vi "read_params.vi"(8 "error in (no error)":errorcluster, 11 "Perceptron in":refnum<class "Perceptron.lvclass">) -> (0 "error out":errorcluster, 2 "params":T1={"penalty"="l2", "alpha"=0.001, "l1_ratio"=0.15, "fit_intercept"=TRUE, "max_iter"=1000.0, "tol"=0.001, "shuffle"=TRUE, "verbose"=0.0, "n_jobs"=1.0, "random_state"=0.0, "early_stopping"=FALSE, "validation_fraction"=0.1, "n_iter_no_change"=5.0, "class_weight"={"class_weight_type"="None", "class_weight_dict"="{0:1.2,1:0.8,2:1.0}"}, "warm_start"=FALSE}, 3 "Perceptron out":refnum<class "Perceptron.lvclass">)   [LabVIEW 2020, in "Perceptron.lvclass"]
uses:
  Perceptron.lvclass
  Controls/perceptron_params.ctl
  Perceptron.lvclass/Perceptron.ctl
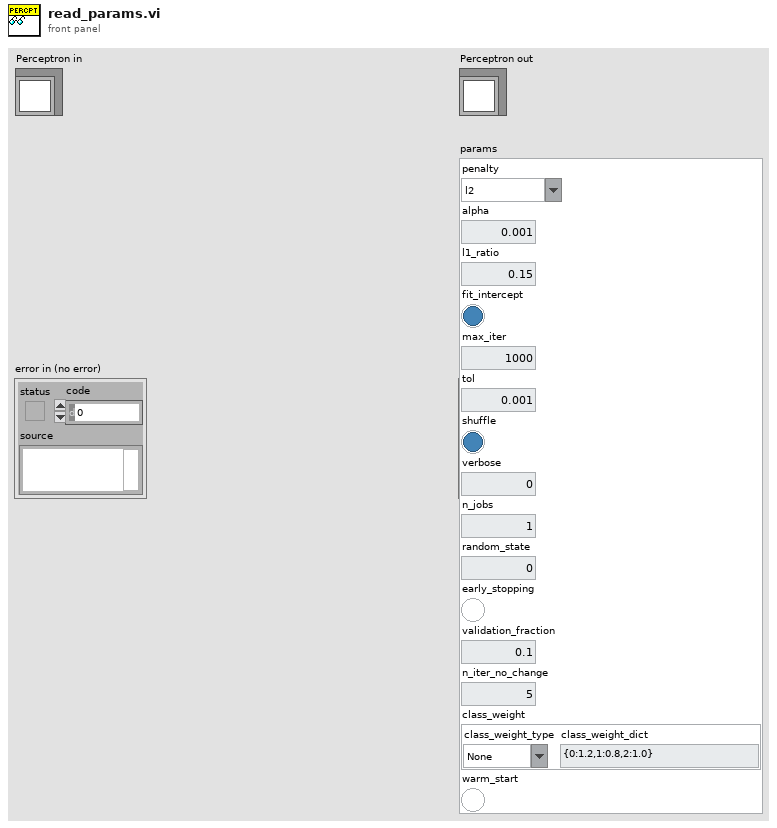
[diagram p1: front panel]
types:
  T1 = typedef "perceptron_params.ctl" = cluster{"penalty":string, "alpha":dbl, "l1_ratio":dbl, "fit_intercept":bool, "max_iter":dbl, "tol":dbl, "shuffle":bool, "verbose":dbl, "n_jobs":dbl, "random_state":dbl, "early_stopping":bool, "validation_fraction":dbl, "n_iter_no_change":dbl, "class_weight":cluster{"class_weight_type":string, "class_weight_dict":string}, "warm_start":bool}
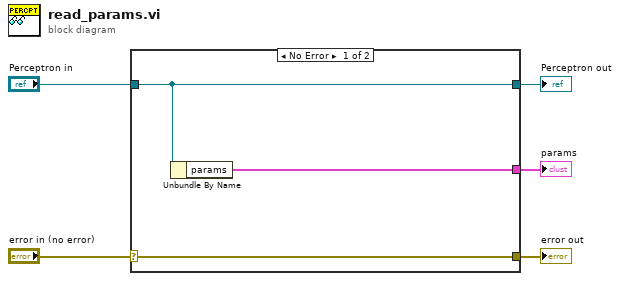
[diagram p0: block diagram]
diagram:
  n1 = case shown="No Error" "error in (no error)" {
    selector: "error in (no error)" -> [w8 w9]
    tunnel: [w8 w9] -> w4
    tunnel: [w7 w10] -> w2
    tunnel: "Perceptron in" -> [w7 w10]
    tunnel: [w6 _] -> w1
    frame No Error {
      n2 = Unbundle By Name(w7) -> ("params"=w6:T1)
    }
    frame Error {
    }
  }
  "error out" <- w4
  "Perceptron out" <- w2
  "params" <- w1
